vi "Weighted_Cross_Moments.vi"(0 "AI Cluster 1":T3={"Colour"=0, "Inst type"=enum."Pitot-static tube", "Inst name"="Manometer voltage", "Symbol"="U", "Code name"="", "Extra Info"="U", "Inst Array"=enum."PWA", "Extra Titles"=[], "Extra Values"=[], "U"=0.0, "u^2"=0.0, "u^3"=0.0, "u^4"=0.0, "Skew_u"=0.0, "Kurt_u"=0.0, "Sd Error in Mean"=0.0, "% u'/U"=0.0, "X"=0.0, "Y"=0.0, "Z"=0.0, "Timescale integral Estimate"=0.0, "Sd Error in Variance"=0.0, "Calib File"=path "", "Calib Constants"=[], "Output Position"=FALSE, "Full Stats"=FALSE, "Av Sampling Rate"=0.0, "Av No of Samples"=0.0, "Total Meas Time (s)"=0.0, "ADAM Ch Name"="", "Max value"=0.0, "Min value"=0.0} {"Sd Error in Variance" format="%.2f"; "Skew_u" format="%.2f"; "% u'/U" format="%.2f"; "Sd Error in Mean" format="%.2f"; "Kurt_u" format="%.2f"; "u^4" format="%.2f"; "u^3" format="%.2f"; "U" format="%.2f"; "u^2" format="%.2f"}, 1 "AI Cluster 2":T3={"Colour"=0, "Inst type"=enum."Pitot-static tube", "Inst name"="Manometer voltage", "Symbol"="U", "Code name"="", "Extra Info"="U", "Inst Array"=enum."PWA", "Extra Titles"=[], "Extra Values"=[], "U"=0.0, "u^2"=0.0, "u^3"=0.0, "u^4"=0.0, "Skew_u"=0.0, "Kurt_u"=0.0, "Sd Error in Mean"=0.0, "% u'/U"=0.0, "X"=0.0, "Y"=0.0, "Z"=0.0, "Timescale integral Estimate"=0.0, "Sd Error in Variance"=0.0, "Calib File"=path "", "Calib Constants"=[], "Output Position"=FALSE, "Full Stats"=FALSE, "Av Sampling Rate"=0.0, "Av No of Samples"=0.0, "Total Meas Time (s)"=0.0, "ADAM Ch Name"="", "Max value"=0.0, "Min value"=0.0} {"Sd Error in Variance" format="%.2f"; "Skew_u" format="%.2f"; "% u'/U" format="%.2f"; "Sd Error in Mean" format="%.2f"; "Kurt_u" format="%.2f"; "u^4" format="%.2f"; "u^3" format="%.2f"; "U" format="%.2f"; "u^2" format="%.2f"}, 2 "Time Cluster 1":T1, 3 "Time Cluster 2":T1, 5 "Shift in":dbl[](array[numeric]) format="%.2f", 9 "interp. method":i32(ring)=1 items=["nearest", "linear", "spline", "cubic Hermite", "Lagrange"]) -> (17 "output cluster":T2 {"Timescale of uw" format="%.2f"; "Sd Error in uw" format="%.2f"; "u^2w^2" format="%.2f"; "u^3w" format="%.2f"; "uw^3" format="%.2f"; "uw/u'w'" format="%.2f"; "uw^2" format="%.2f"; "u^2w" format="%.2f"; "uw" format="%.2f"}, 19 "Shift out":dbl[](array[numeric]) format="%.2f")   [LabVIEW 2016]
uses:
  Controls/Analysis_info_cluster.ctl
  Controls/Inst_type.ctl
  Controls/Instrument_Array.ctl
  Controls/Correlation_cluster1.ctl
  Controls/Time_Trace_Cluster.ctl
  Globals/Meas_global.vi
  <vilib>/gmath/NI_Gmath.lvlib
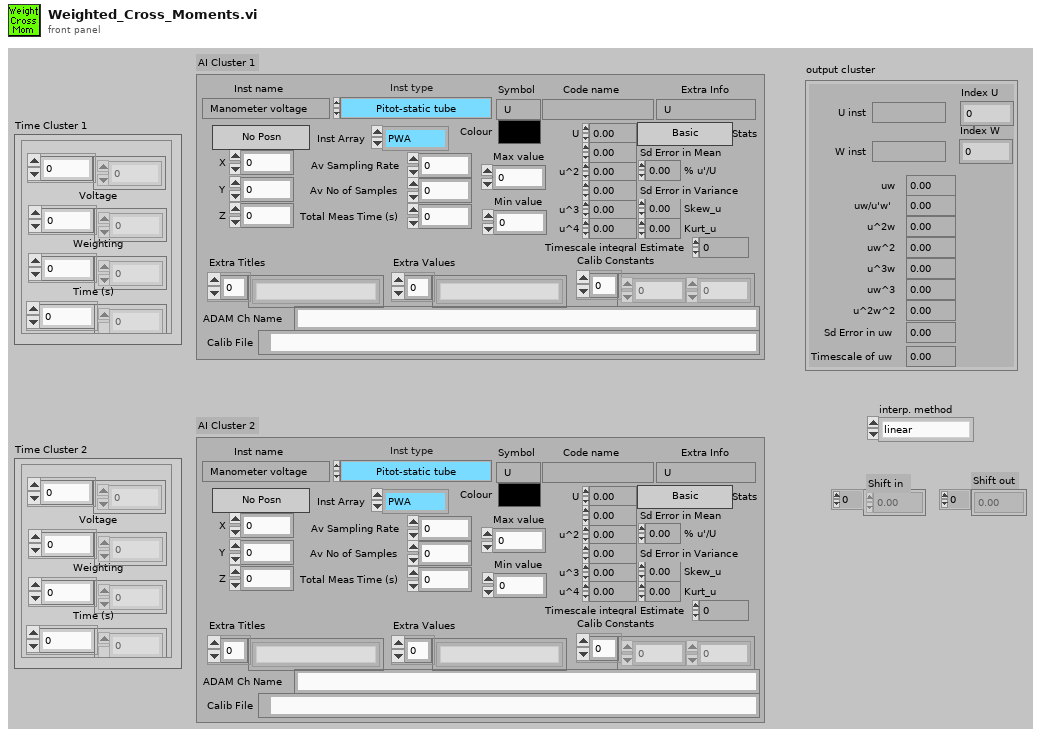
[diagram p1: front panel]
types:
  T1 = typedef "Time_Trace_Cluster.ctl" = cluster{"Weighting":dbl[], "Time (s)":dbl[], "Voltage":dbl[], "Eng Values":dbl[]}
  T2 = typedef "Correlation_cluster1.ctl" = cluster{"U inst":string, "uw":dbl, "u^2w":dbl, "uw^2":dbl, "uw/u'w'":dbl, "W inst":string, "uw^3":dbl, "u^3w":dbl, "u^2w^2":dbl, "Index U":i32, "Index W":i32, "Sd Error in uw":dbl, "Timescale of uw":dbl}
  T3 = typedef "Analysis_info_cluster.ctl" = cluster{"Colour":u32, "Inst type":T4, "Inst name":string, "Symbol":string, "Code name":string, "Extra Info":string, "Inst Array":T5, "Extra Titles":string[], "Extra Values":string[], "U":dbl, "u^2":dbl, "u^3":dbl, "u^4":dbl, "Skew_u":dbl, "Kurt_u":dbl, "Sd Error in Mean":dbl, "% u'/U":dbl, "X":dbl, "Y":dbl, "Z":dbl, "Timescale integral Estimate":dbl, "Sd Error in Variance":dbl, "Calib File":path, "Calib Constants":dbl[], "Output Position":bool, "Full Stats":bool, "Av Sampling Rate":dbl, "Av No of Samples":dbl, "Total Meas Time (s)":dbl, "ADAM Ch Name":string, "Max value":dbl, "Min value":dbl}
  T4 = typedef "Inst_type.ctl" = enum16{"Propeller anemometer", "Raw voltage", "Pressure Transducer", "Pitot-static tube", "Preston tube", "Hot wire", "Cross wire 1", "Cross wire 2", "Generic Linear", "Generic Polynomial", "Generic BackPoly", "Fast FID", "Thermocouple", "Cold wire", "Pulsed Wire", "LDA Vel", "LDA Tran time", "LDA Arr time", "Microphone"}
  T5 = typedef "Instrument_Array.ctl" = enum16{"PWA", "LDA", "Analogue"}
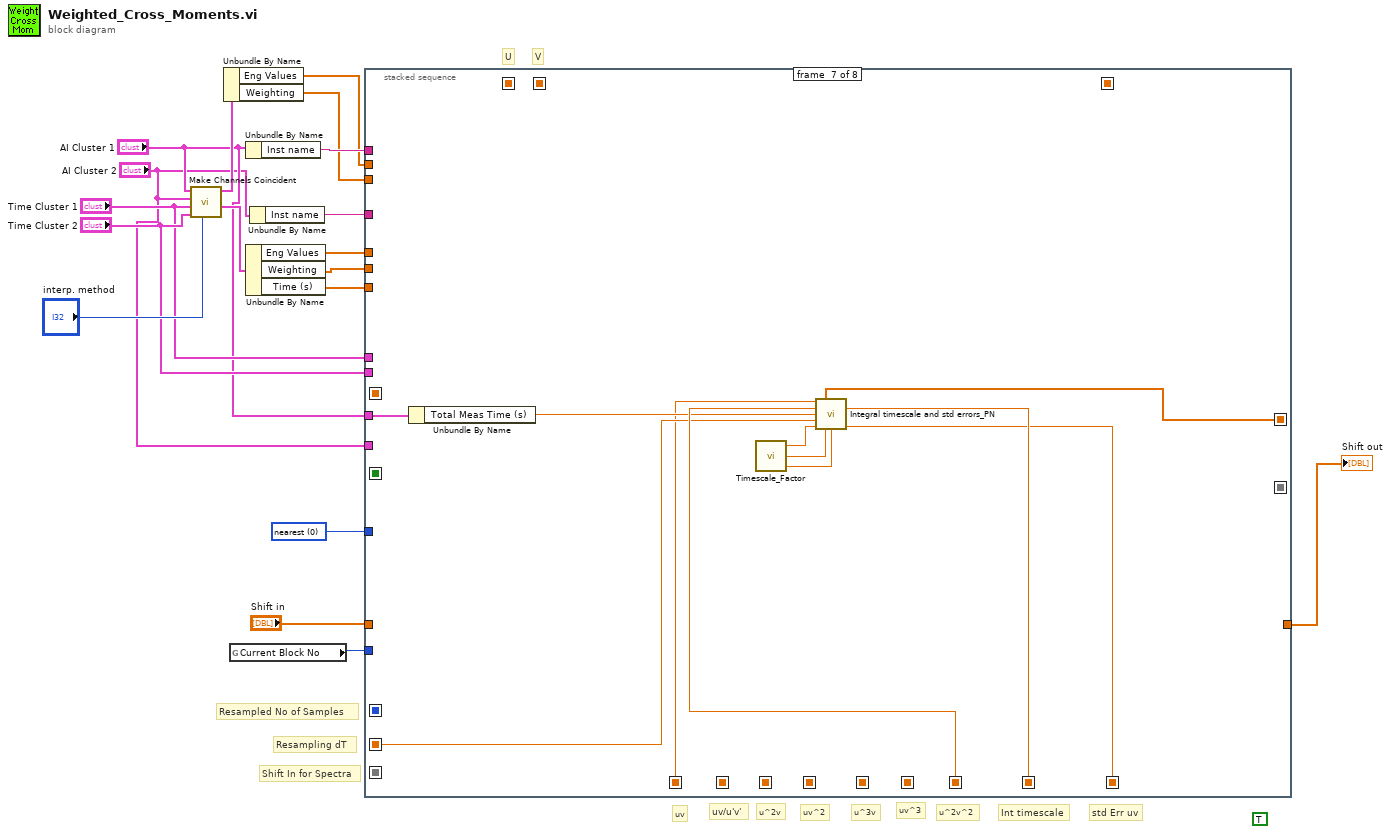
[diagram p0: block diagram]
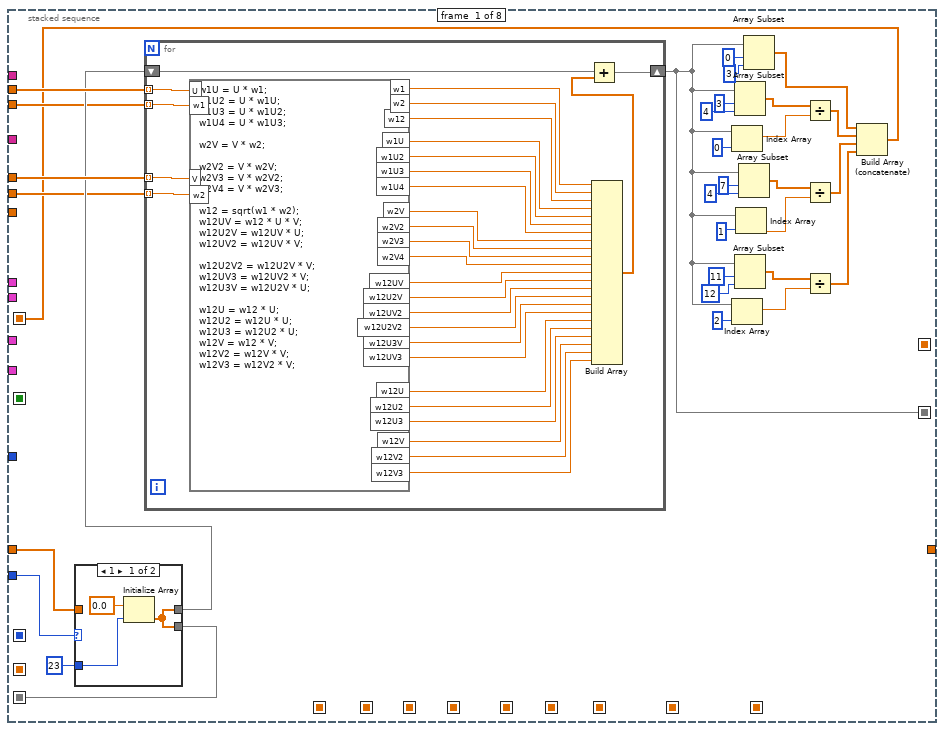
[diagram p2: hidden frame]
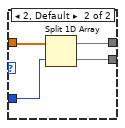
[diagram p3: hidden frame]
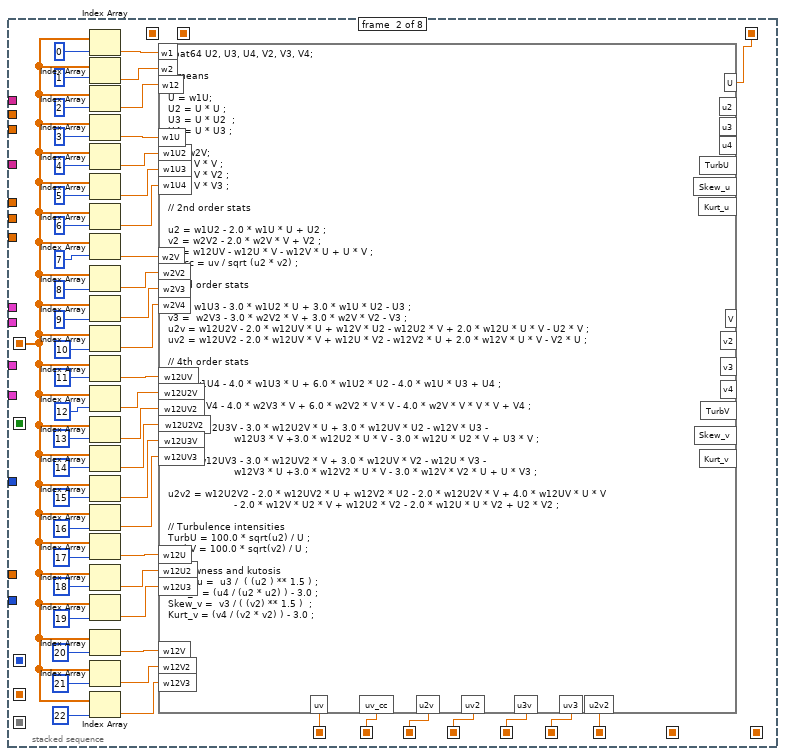
[diagram p4: hidden frame]
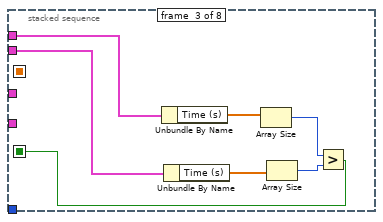
[diagram p5: hidden frame]
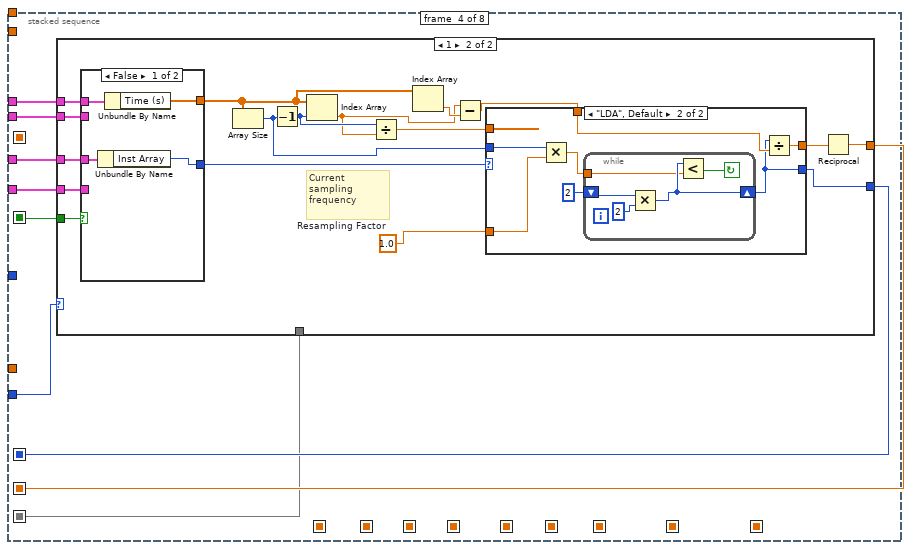
[diagram p6: hidden frame]
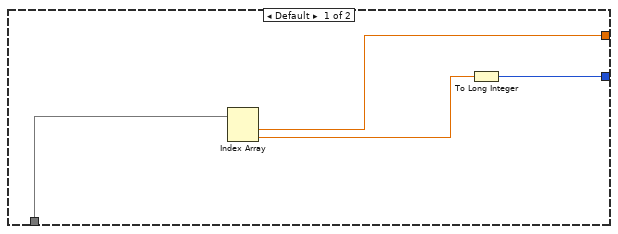
[diagram p7: hidden frame]
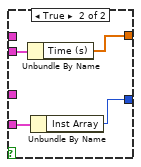
[diagram p9: hidden frame]
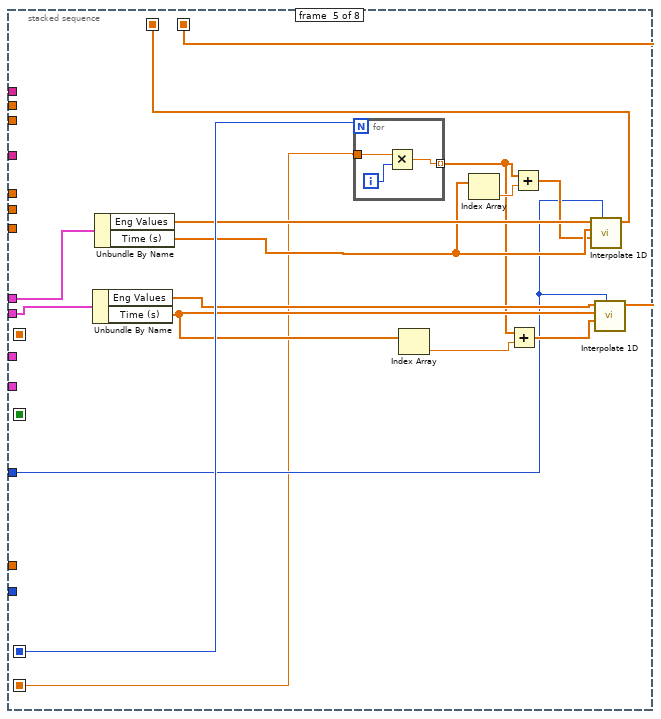
[diagram p10: hidden frame]
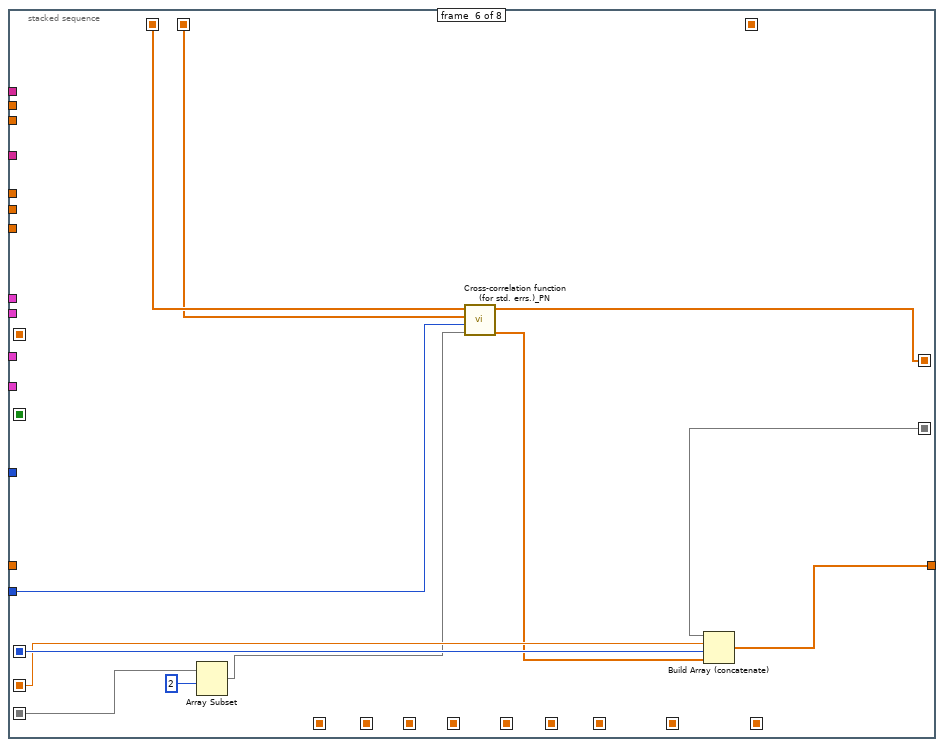
[diagram p11: hidden frame]
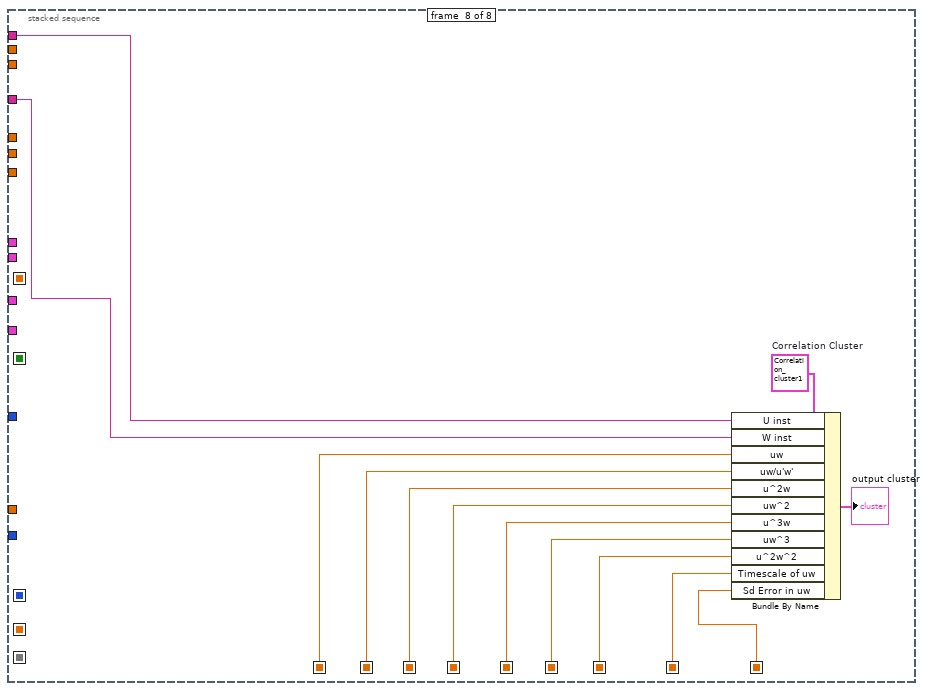
[diagram p12: hidden frame]
diagram:
  w1 = 0 items=["nearest", "linear", "spline", "cubic Hermite", "Lagrange"] ("method")
  (unwired) TRUE
  # "Int timescale"
  # "std Err uv"
  # "V"
  # "U"
  # "Shift In for Spectra"
  # "Resampling dT"
  # "Resampled No of Samples"
  # "u^2v^2"
  # "uv^3"
  # "u^3v"
  # "uv^2"
  # "u^2v"
  # "uv/u'v'"
  # "uv"
  n1 = call "Make Channels Coincident.vi"("interp. method"="interp. method", "Time Cluster 2"="Time Cluster 2", "Time Cluster 1"="Time Cluster 1", "Cluster 2"="AI Cluster 2", "Cluster 1"="AI Cluster 1") -> ("Coincident Time Cluster 2"=w7:T1, "Coincident Time Cluster 1"=w8:T1)  [unwired: 5 in]
  n2 = Unbundle By Name(w8) -> ("Eng Values"=w13:dbl[], "Weighting"=w12:dbl[])
  n3 = global read "Meas_global.vi" "Current Block No"() -> (w16:i32)
  n4 = Unbundle By Name("AI Cluster 1") -> ("Inst name"=w18:string)
  n5 = Unbundle By Name(w7) -> ("Eng Values"=w11:dbl[], "Weighting"=w10:dbl[], "Time (s)"=w6:dbl[])
  n6 = Unbundle By Name("AI Cluster 2") -> ("Inst name"=w17:string)
  n7 = stacked-sequence {
    seq-local: [_ w130 _ _ _ _ _ _] -> [_ _ _ _ _ _ w237 w253]
    seq-local: [_ w129 _ _ _ _ _ _] -> [_ _ _ _ _ _ _ w252]
    seq-local: [w43 _ _ _ _ _ _ _] -> [_ w91 _ _ _ _ _ _]
    seq-local: [_ w124 _ _ _ _ _ _] -> [_ _ _ _ _ _ _ w251]
    seq-local: [_ w123 _ _ _ _ _ _] -> [_ _ _ _ _ _ _ w250]
    seq-local: [_ w104 _ _ _ _ _ _] -> [_ _ _ _ _ _ _ w249]
    seq-local: [_ w103 _ _ _ _ _ _] -> [_ _ _ _ _ _ _ w248]
    seq-local: [_ w102 _ _ _ _ _ _] -> [_ _ _ _ _ _ w242 w247]
    seq-local: [_ _ w143 _ _ _ _ _] -> [_ _ _ w158 _ _ _ _]
    seq-local: [_ _ _ w153 _ _ _ _] -> [_ _ _ _ w217 w228 _ _]
    seq-local: [_ _ _ w152 _ _ _ _] -> [_ _ _ _ w202 w227 w241 _]
    seq-local: [w20 _ _ _ _ _ _ _] -> [_ _ _ w150 _ w231 _ _]
    seq-local: [_ _ _ _ w211 _ _ _] -> [_ _ _ _ _ w222 _ _]
    seq-local: [_ _ _ _ w203 _ _ _] -> [_ _ _ _ _ w221 _ _]
    seq-local: [w19 _ _ _ _ _ _ _] -> [_ _ _ _ _ w230 _ _]
    seq-local: [_ w88 _ _ _ _ _ _] -> [_ _ _ _ _ _ _ _]
    seq-local: [_ _ _ _ _ w223 _ _] -> [_ _ _ _ _ _ w243 _]
    seq-local: [_ _ _ _ _ _ w236 _] -> [_ _ _ _ _ _ _ w244]
    seq-local: [_ _ _ _ _ _ w240 _] -> [_ _ _ _ _ _ _ w245]
    tunnel: w13 -> [w50 _ _ _ _ _ _ _]
    tunnel: "Shift in" -> [w47 _ _ _ _ _ _ _]
    tunnel: w11 -> [w49 _ _ _ _ _ _ _]
    tunnel: w16 -> [w48 _ _ w151 _ w225 _ _]
    tunnel: w12 -> [w45 _ _ _ _ _ _ _]
    tunnel: w10 -> [w44 _ _ _ _ _ _ _]
    tunnel: w18 -> [_ _ _ _ _ _ _ w255]
    tunnel: w17 -> [_ _ _ _ _ _ _ w254]
    tunnel: [_ _ _ _ _ w229 _ _] -> w15
    tunnel: w6 -> [_ _ _ _ _ _ _ _]
    tunnel: "Time Cluster 2" -> [_ _ w147 w157 w210 _ _ _]
    tunnel: "Time Cluster 1" -> [_ _ w146 w156 w216 _ _ _]
    tunnel: "AI Cluster 1" -> [_ _ _ w155 _ _ w239 _]
    tunnel: "AI Cluster 2" -> [_ _ _ w154 _ _ _ _]
    tunnel: w1 -> [_ _ _ _ w204 _ _ _]
    frame #0 {
      n8 = case shown="1" w48 {
        tunnel: [w51 w55] -> w46
        tunnel: w47 -> [_ w56]
        tunnel: 23 ("Dimension Size") -> [w52 w57]
        tunnel: [w51 w54] -> w20
        frame 1 {
          n9 = Initialize Array(0.0 ("Element Data"), w52) -> (w51:dbl[])
        }
        frame 2, Default {
          n10 = Split 1D Array(array=w56, index=w57) -> (first subarray=w55:dbl[], second subarray=w54:dbl[])
        }
      }
      n11 = for {
        shift-right: [w83] -> w19
        shift-left: w46 -> [w87]
        tunnel: w45 -> [w82] mode=indexing
        tunnel: w50 -> [w85] mode=indexing
        tunnel: w49 -> [w84] mode=indexing
        tunnel: w44 -> [w81] mode=indexing
        n12 = formula code="w1U = U * w1;\nw1U2 = U * w1U;\nw1U3 = U * w1U2;\nw1U4 = U * w1U3;\n\nw2V = V * w2;\n\nw2V2 = V * w2V;\nw2V3 = V * w2V2;\nw2V4 = V * w2V3;\n\nw12 = sqrt(w1 * w2);\nw12UV = w12 * U * V;\nw12U2V = w12UV * U;\nw12UV2 = w12UV * V;\n\nw12U2V2 = w12U2V * V;\nw12UV3 = w12UV2 * V;\nw12U3V = w12U2V * U;\n\nw12U = w12 * U;\nw12U2 = w12U * U;\nw12U3 = w12U2 * U;\nw12V = w12 * V;\nw12V2 = w12V * V;\nw12V3 = w12V2 * V;"("V"=w84, "U"=w85, "w1"=w82, "w2"=w81) -> ("w12UV"=w72:dbl, "w1U"=w80:dbl, "w2V"=w76:dbl, "w1U2"=w79:dbl, "w2V2"=w75:dbl, "w12U2V"=w71:dbl, "w12UV2"=w70:dbl, "w1U3"=w78:dbl, "w1U4"=w77:dbl, "w2V3"=w74:dbl, "w2V4"=w73:dbl, "w12U3V"=w68:dbl, "w12UV3"=w67:dbl, "w12U2V2"=w69:dbl, "w12U"=w63:dbl, "w12U2"=w62:dbl, "w12U3"=w61:dbl, "w12V"=w60:dbl, "w12V2"=w59:dbl, "w12V3"=w58:dbl, "w12"=w66:dbl, "w1"=w65:dbl, "w2"=w64:dbl)
        n13 = Build Array(w65, w64, w66, w80, w79, w78, w77, w76, w75, w74, w73, w72, w71, w70, w69, w68, w67, w63, w62, w61, w60, w59, w58) -> (w86:dbl[])
        n14 = Add(x=w87, y=w86) -> (x+y=w83:dbl[])
      }
      n15 = Index Array(array=w19, index=0 ("Index")) -> (element=w39:dbl)
      n16 = Index Array(array=w19, index=2 ("Index")) -> (element=w29:dbl)
      n17 = Array Subset(array=w19, index=3 ("Array Index"), length=4) -> (w40:dbl[])
      n18 = Array Subset(array=w19, index=11 ("Array Index"), length=12) -> (w30:dbl[])
      n19 = Index Array(array=w19, index=1 ("Index")) -> (element=w36:dbl)
      n20 = Array Subset(array=w19, index=7 ("Array Index"), length=4) -> (w35:dbl[])
      n21 = Array Subset(array=w19, index=0, length=3) -> (w22:dbl[])
      n22 = Divide(x=w40, y=w39) -> (x/y=w27:dbl[])
      n23 = Divide(x=w35, y=w36) -> (x/y=w26:dbl[])
      n24 = Divide(x=w30, y=w29) -> (x/y=w25:dbl[])
      n25 = Build Array (concatenate)(w22, w27, w26, w25) -> (w43:dbl[])
    }
    frame #1 {
      n26 = Index Array(array=w91, index=0) -> (element=w136:dbl)
      n27 = Index Array(array=w91, index=1) -> (element=w135:dbl)
      n28 = Index Array(array=w91, index=2) -> (element=w134:dbl)
      n29 = Index Array(array=w91, index=3) -> (element=w133:dbl)
      n30 = Index Array(array=w91, index=4) -> (element=w132:dbl)
      n31 = Index Array(array=w91, index=5) -> (element=w131:dbl)
      n32 = Index Array(array=w91, index=6) -> (element=w126:dbl)
      n33 = Index Array(array=w91, index=7) -> (element=w125:dbl)
      n34 = Index Array(array=w91, index=8) -> (element=w116:dbl)
      n35 = Index Array(array=w91, index=9) -> (element=w115:dbl)
      n36 = Index Array(array=w91, index=10) -> (element=w118:dbl)
      n37 = Index Array(array=w91, index=11) -> (element=w117:dbl)
      n38 = Index Array(array=w91, index=12) -> (element=w112:dbl)
      n39 = Index Array(array=w91, index=13) -> (element=w111:dbl)
      n40 = Index Array(array=w91, index=14) -> (element=w107:dbl)
      n41 = Index Array(array=w91, index=15) -> (element=w106:dbl)
      n42 = Index Array(array=w91, index=16) -> (element=w105:dbl)
      n43 = Index Array(array=w91, index=17) -> (element=w97:dbl)
      n44 = Index Array(array=w91, index=18) -> (element=w96:dbl)
      n45 = Index Array(array=w91, index=19) -> (element=w95:dbl)
      n46 = Index Array(array=w91, index=20) -> (element=w94:dbl)
      n47 = Index Array(array=w91, index=21) -> (element=w90:dbl)
      n48 = Index Array(array=w91, index=22) -> (element=w89:dbl)
      n49 = formula code="float64 U2, U3, U4, V2, V3, V4;\n\n// means\n\nU = w1U;\nU2 = U * U ;\nU3 = U * U2  ;\nU4 = U * U3 ;\n\nV = w2V;\nV2 = V * V ;\nV3 = V * V2 ;\nV4 = V * V3 ;\n\n// 2nd order stats\n\nu2 = w1U2 - 2.0 * w1U * U + U2 ;\nv2 = w2V2 - 2.0 * w2V * V + V2 ;\nuv = w12UV - w12U * V - w12V * U + U * V ;\nuv_cc = uv / sqrt (u2 * v2) ;\n\n// 3rd order stats\n\nu3 = w1U3 - 3.0 * w1U2 * U + 3.0 * w1U * U2 - U3 ;\nv3 =  w2V3 - 3.0 * w2V2 * V + 3.0 * w2V * V2 - V3 ;\nu2v = w12U2V - 2.0 * w12UV * U + w12V * U2 - w12U2 * V + 2.0 * w12U * U * V - U2 * V ;\nuv2 = w12UV2 - 2.0 * w12UV * V + w12U * V2 - w12V2 * U + 2.0 * w12V * U * V - V2 * U ;\n\n// 4th order stats\n\nu4 = w1U4 - 4.0 * w1U3 * U + 6.0 * w1U2 * U2 - 4.0 * w1U * U3 + U4 ;\n\nv4 = w2V4 - 4.0 * w2V3 * V + 6.0 * w2V2 * V * V - 4.0 * w2V * V * V * V + V4 ;\n\nu3v = w12U3V - 3.0 * w12U2V * U + 3.0 * w12UV * U2 - w12V * U3 - \n                      w12U3 * V +3.0 * w12U2 * U * V - 3.0 * w12U * U2 * V + U3 * V ;\n\nuv3 = w12UV3 - 3.0 * w12UV2 * V + 3.0 * w12UV * V2 - w12U * V3 - \n                      w12V3 * U +3.0 * w12V2 * U * V - 3.0 * w12V * V2 * U + U * V3 ;\n\nu2v2 = w12U2V2 - 2.0 * w12UV2 * U + w12V2 * U2 - 2.0 * w12U2V * V + 4.0 * w12UV * U * V\n                      - 2.0 * w12V * U2 * V + w12U2 * V2 - 2.0 * w12U * U * V2 + U2 * V2 ; \n\n// Turbulence intensities\nTurbU = 100.0 * sqrt(u2) / U ;\nTurbV = 100.0 * sqrt(v2) / U ;\n\n// Skewness and kutosis\nSkew_u =  u3 /  ( (u2 ) ** 1.5 ) ;\nKurt_u = (u4 / (u2 * u2) ) - 3.0 ;\nSkew_v =  v3 / ( (v2) ** 1.5 )  ;\nKurt_v = (v4 / (v2 * v2) ) - 3.0 ;"("w1"=w136, "w2"=w135, "w12"=w134, "w1U2"=w132, "w1U3"=w131, "w1U"=w133, "w1U4"=w126, "w2V"=w125, "w2V2"=w116, "w2V4"=w118, "w2V3"=w115, "w12UV"=w117, "w12U2V"=w112, "w12UV2"=w111, "w12U2V2"=w107, "w12U3V"=w106, "w12UV3"=w105, "w12U2"=w96, "w12U3"=w95, "w12V"=w94, "w12V2"=w90, "w12U"=w97, "w12V3"=w89) -> ("uv"=w130:dbl, "U"=w88:dbl, "uv_cc"=w129:dbl, "u2v"=w124:dbl, "uv2"=w123:dbl, "u3v"=w104:dbl, "uv3"=w103:dbl, "u2v2"=w102:dbl)  [unwired: 13 out]
    }
    frame #2 {
      n50 = Unbundle By Name(w146) -> ("Time (s)"=w145:dbl[])
      n51 = Unbundle By Name(w147) -> ("Time (s)"=w144:dbl[])
      n52 = Array Size(array=w145) -> (size(s)=w149:i32)
      n53 = Array Size(array=w144) -> (size(s)=w148:i32)
      n54 = Greater?(x=w149, y=w148) -> (0:w143:bool)
    }
    frame #3 {
      n55 = case shown="1" w151 {
        tunnel: w158 -> [_ w179]
        tunnel: w157 -> [_ w178]
        tunnel: w156 -> [_ w176]
        tunnel: w155 -> [_ w175]
        tunnel: w154 -> [_ w174]
        tunnel: [w159 w172] -> w153
        tunnel: [w161 w163] -> w152
        tunnel: w150 -> [w162 _]
        frame Default {
          n56 = Index Array(array=w162) -> (element #1=w161:dbl, element #2=w160:dbl)  [unwired: 2 in]
          n57 = To Long Integer(number=w160) -> (32bit integer=w159:i32)
        }
        frame 1 {
          w168 = 1.0  # Resampling Factor
          # "Current sampling\nfrequency"
          n58 = case shown="False" w179 {
            tunnel: w178 -> [_ w201]
            tunnel: [w196 w200] -> w177
            tunnel: w176 -> [w197 _]
            tunnel: w175 -> [w195 _]
            tunnel: w174 -> [_ w199]
            tunnel: [w194 w198] -> w173
            frame False {
              n59 = Unbundle By Name(w195) -> ("Inst Array"=w194:T5)
              n60 = Unbundle By Name(w197) -> ("Time (s)"=w196:dbl[])
            }
            frame True {
              n61 = Unbundle By Name(w201) -> ("Time (s)"=w200:dbl[])
              n62 = Unbundle By Name(w199) -> ("Inst Array"=w198:T5)
            }
          }
          n63 = Array Size(array=w177) -> (size(s)=w169:i32)
          n64 = Decrement(x=w169) -> (x-1=w170:i32)
          n65 = Index Array(array=w177, index=w170) -> (element=w165:dbl)
          n66 = Divide(x=w170, y=w165) -> (x/y=w171:dbl)
          n67 = Index Array(array=w177) -> (element=w167:dbl)  [unwired: 1 in]
          n68 = Subtract(x=w165, y=w167) -> (x-y=w166:dbl)
          n69 = case shown="\"LDA\", Default" w173 {
            tunnel: w171 -> [w181 _]
            tunnel: w166 -> [_ w188]
            tunnel: [w181 w187] -> w164
            tunnel: w169 -> [w180 w185]
            tunnel: [w180 w184] -> w172
            tunnel: w168 -> [_ w183]
            frame "Analogue" {
            }
            frame "LDA", Default {
              n70 = Multiply(x=w185, y=w183) -> (x*y=w186:dbl)
              n71 = while {
                shift-right: [w191] -> w184
                shift-left: 2 -> [w193]
                tunnel: w186 -> [w189]
                stop <- w190 continue-if-true
                n72 = Multiply(x=w193, y=2) -> (x*y=w191:i32)
                n73 = Less?(x=w191, y=w189) -> (x < y?=w190:bool)
              }
              n74 = Divide(x=w184, y=w188) -> (x/y=w187:dbl)
            }
          }
          n75 = Reciprocal(x=w164) -> (1/x=w163:dbl)
        }
      }
    }
    frame #4 {
      n76 = Unbundle By Name(w210) -> ("Eng Values"=w209:dbl[], "Time (s)"=w208:dbl[])
      n77 = Unbundle By Name(w216) -> ("Eng Values"=w215:dbl[], "Time (s)"=w214:dbl[])
      n78 = for {
        N: w217 -> [_]
        tunnel: w202 -> [w220]
        tunnel: [w218] -> w207 mode=indexing
        i -> [w219]
        n79 = Multiply(x=w220, y=w219) -> (x*y=w218:dbl)
      }
      n80 = Index Array(array=w208) -> (element=w206:dbl)  [unwired: 1 in]
      n81 = Index Array(array=w214) -> (element=w213:dbl)  [unwired: 1 in]
      n82 = Add(x=w207, y=w206) -> (x+y=w205:dbl[])
      n83 = Add(x=w207, y=w213) -> (x+y=w212:dbl[])
      n84 = call <vilib>:"Interpolate 1D.vi"("method"=w204, "xi"=w212, "X"=w214, "Y"=w215) -> ("yi"=w211:dbl[])  [unwired: 2 in, 5 out]
      n85 = call <vilib>:"Interpolate 1D.vi"("method"=w204, "xi"=w205, "X"=w208, "Y"=w209) -> ("yi"=w203:dbl[])  [unwired: 2 in, 5 out]
    }
    frame #5 {
      n86 = Array Subset(array=w231, index=2) -> (w226:dbl[])  [unwired: 1 in]
      n87 = call "Cross-correlation function (for std. errs.)_PN.vi"("Shift in"=w226, "Current Block No"=w225, "V (m/s)"=w221, "U (m/s)"=w222) -> ("Shift Out"=w224:dbl[], "Cross-correlation function"=w223:dbl[])  [unwired: 2 in]
      n88 = Build Array (concatenate)(w230, w227, w228, w224) -> (w229:dbl[])
    }
    frame #6 {
      n89 = Unbundle By Name(w239) -> ("Total Meas Time (s)"=w238:dbl)
      n90 = call "Timescale_Factor.vi"() -> ("Timescale multiplier for independent samples"=w233:dbl, "Timescale scaling factor"=w235:dbl, "Integration threshold (0...1)"=w234:dbl)  [unwired: 3 in]
      n91 = call "Integral timescale and std errors_PN.vi"("uv_bar (m/s)^2"=w237, "Cross-correlation function"=w243, "u2v2_bar (m/s)^4"=w242, "T_meas (s)"=w238, "dt (s)"=w241, "integral cut-off"=w234, "integral post-mult"=w235, "Timescale multiple for independent samples"=w233) -> ("Integral timescale (s)"=w240:dbl, "Std. err in uv (m/s^2)"=w236:dbl)  [unwired: 4 in, 2 out]
    }
    frame #7 {
      w256 = T2 {"U inst"="", "uw"=0.0, "u^2w"=0.0, "uw^2"=0.0, "uw/u'w'"=0.0, "W inst"="", "uw^3"=0.0, "u^3w"=0.0, "u^2w^2"=0.0, "Index U"=0, "Index W"=0, "Sd Error in uw"=0.0, "Timescale of uw"=0.0}  # Correlation Cluster
      n92 = Bundle By Name(cluster=w256, "U inst"=w255, "W inst"=w254, "uw"=w253, "uw/u'w'"=w252, "u^2w"=w251, "uw^2"=w250, "u^3w"=w249, "uw^3"=w248, "u^2w^2"=w247, "Timescale of uw"=w245, "Sd Error in uw"=w244) -> (→"output cluster":T2)
    }
  }
  "Shift out" <- w15
